vi "set Menu Visible.vi"(8 "error in (no error)":errorcluster, 10 "Menu Visible":bool, 11 "Actor in":refnum<class "Actor.lvclass">) -> (0 "error out":errorcluster, 3 "Actor out":refnum<class "Actor.lvclass">)   [LabVIEW 2015, in "Actor.lvclass"]
uses:
  Actor.lvclass
  Actor.lvclass/Actor.ctl
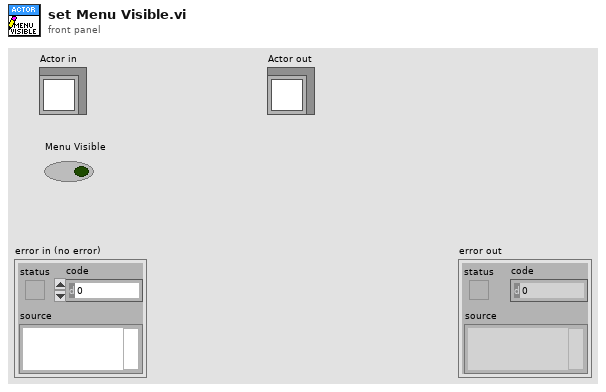
[diagram p1: front panel]
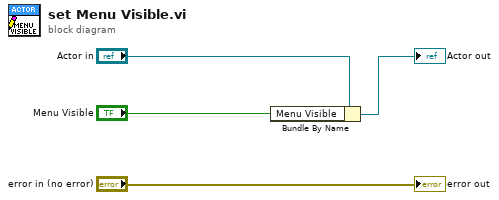
[diagram p0: block diagram]
diagram:
  n1 = Bundle By Name(cluster="Actor in", "Menu Visible"="Menu Visible") -> (→"Actor out":refnum<class "Actor.lvclass">)
  "error out" <- "error in (no error)"
